vi "Manual Shooter Speed.vi"(10 "Buttons":bool[](array[boolean]), 11 "%Vbus Increments":dbl=0.05 format="%#_13g") -> (1 "Get to Speed?":bool, 2 "Shoot?":bool, 3 "Shooter %Vbus":dbl)   [LabVIEW 2015]
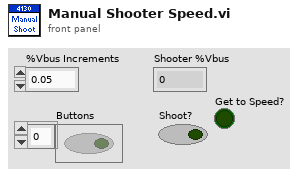
[diagram p1: front panel]
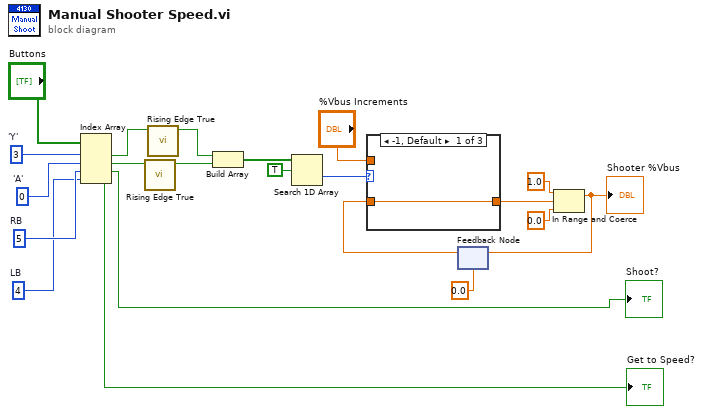
[diagram p0: block diagram]
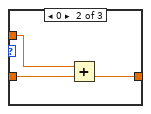
[diagram p2: hidden frame]
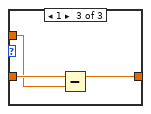
[diagram p3: hidden frame]
diagram:
  w2 = 4  # LB
  w19 = 0  # 'A'
  w18 = 3  # 'Y'
  w16 = 5  # RB
  n1 = Index Array(array="Buttons", index #1=w18, index #2=w19, index #3=w16, index #4=w2) -> (element #1=w9:bool, element #2=w10:bool, element #3=→"Shoot?":bool, element #4=→"Get to Speed?":bool)
  n2 = call "Rising Edge True.vi"("Input"=w10) -> ("Output"=w21:bool)  [unwired: 10 in]
  n3 = call "Rising Edge True.vi"("Input"=w9) -> ("Output"=w20:bool)  [unwired: 10 in]
  n4 = Build Array(w20, w21) -> (w11:bool[])
  n5 = Search 1D Array(1D array=w11, element=TRUE) -> (index of element=w13:i32)  [unwired: 1 in]
  n6 = feedback #1(0.0 ("lower limit")) -> (w7:dbl)
  n7 = case shown="-1, Default" w13 {
    tunnel: w7 -> [w22 w25 w28]
    tunnel: [w22 w24 w27] -> w8
    tunnel: "%Vbus Increments" -> [_ w23 w26]
    frame -1, Default {
    }
    frame 0 {
      n8 = Add(x=w23, y=w25) -> (x+y=w24:dbl)
    }
    frame 1 {
      n9 = Subtract(x=w28, y=w26) -> (x-y=w27:dbl)
    }
  }
  n10 = In Range and Coerce(upper limit=1.0, x=w8, lower limit=0.0) -> (coerced(x)=w15:dbl)  [unwired: 1 out]
  "Shooter %Vbus" <- w15
  n11 = feedback-in #1(w15) -> ()
